vi "rs3 get device.vi"(8 "error in":errorcluster, 10 "index":u32, 11 "context":u32) -> (0 "error out":errorcluster, 2 "device":u32, 3 "context":u64)   [LabVIEW 2023]
doc: "Get the device handle needed for indexed device."
panel:
  # "RS3 Get Device"
  # "(C) Intel Corp.,  AGJ"
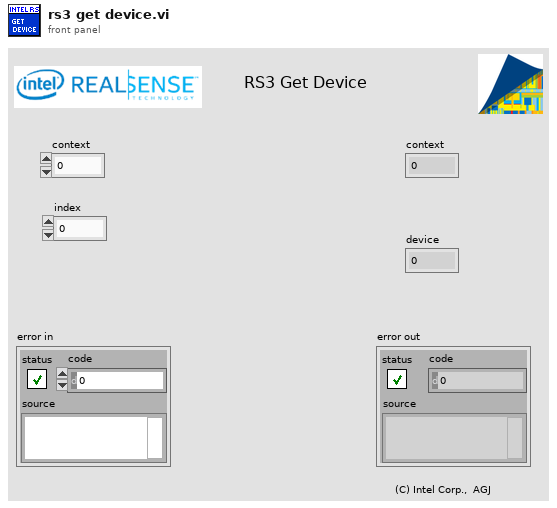
[diagram p1: front panel]
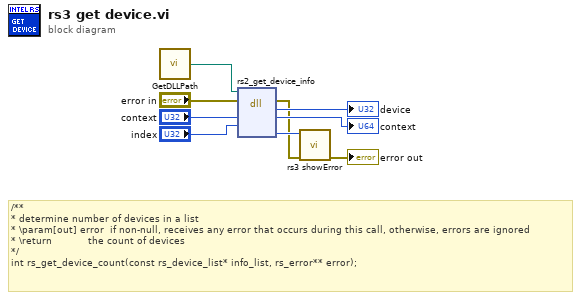
[diagram p0: block diagram]
diagram:
  # "/**\n* determine number of devices in a list\n* \\param[out] error  if non-null, receives any error that occurs during this call, otherwise, errors are ignored\n* \\return            the count of devices\n*/\nint rs_get_device_count(const rs_device_list* info_list, rs_error** error);"
  n1 = call "GetDLLPath.vi"() -> ("DLL Path"=w1:path)
  n2 = dll-call lib="C:/STEAMSyndicate/RealSenseWrappers/VI Wrappers (add ons) Public/RealSense/realsense2.dll" fn="rs2_get_device_info"(path in=w1, error in="error in", "cxt"="context", "id"="index") -> (error out=w3:errorcluster, "device"=→"device":u32, "cxt"=→"context":u64, "error"=w4:u64)  [unwired: 3 in, 1 out]
  n3 = call "rs3 showError.vi"("error in (no error)"=w3, "error"=w4) -> ("error out"=→"error out":errorcluster)  [unwired: 5 in, 4 out]
